vi "AutoDelay.vi"(9 "Delay":dbl) -> ()   [LabVIEW 2020]
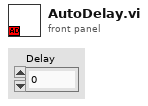
[diagram p1: front panel]
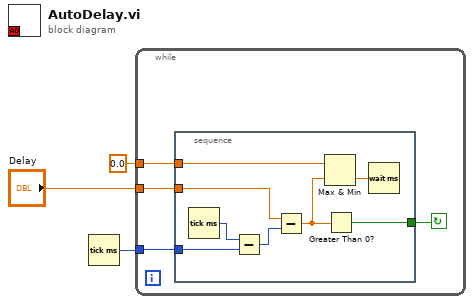
[diagram p0: block diagram]
diagram:
  n1 = Tick Count (ms)() -> (millisecond timer value=w3:u32)
  n2 = while {
    tunnel: "Delay" -> [w5]
    tunnel: 0.0 -> [w6]
    tunnel: w3 -> [w7]
    stop <- w4 continue-if-true
    n3 = stacked-sequence {
      tunnel: w7 -> [w15]
      tunnel: w6 -> [w14]
      tunnel: w5 -> [w12]
      tunnel: [w8] -> w4
      frame #0 {
        n4 = Tick Count (ms)() -> (millisecond timer value=w10:u32)
        n5 = Subtract(x=w10, y=w15) -> (x-y=w11:u32)
        n6 = Subtract(x=w12, y=w11) -> (x-y=w9:dbl)
        n7 = Max & Min(x=w14, y=w9) -> (min(x,y)=w13:dbl)  [unwired: 1 out]
        n8 = Greater Than 0?(x=w9) -> (x > 0?=w8:bool)
        n9 = Wait (ms)(milliseconds to wait=w13) -> ()  [unwired: 1 out]
      }
    }
  }
